vi "duel_ver.vi"() -> ()   [LabVIEW 2024]
uses:
  <vilib>/numeric/Random Number (Range) U64.vi
  <vilib>/numeric/sub_Random U32.vi
panel:
  out "電腦得分":u32
  out "消除數":u16
  out "玩家得分":u32
  out "blocks left":u8
  out "Preview":picture
  in  "Next block":bool
  out "cur block":u8
  out "buf block type":u8[](array[numeric])
  out "rng array":u8[][](array[numeric])
  out "待放置方塊":picture
  in  "direction":enum16{"up", "right", "down", "left"}(ring)
  out "Plate array":u8[][](array[numeric])
  in  "choose_block":u16
  in  "stop":bool
  out "plate":picture
  in  "Turn Block":bool
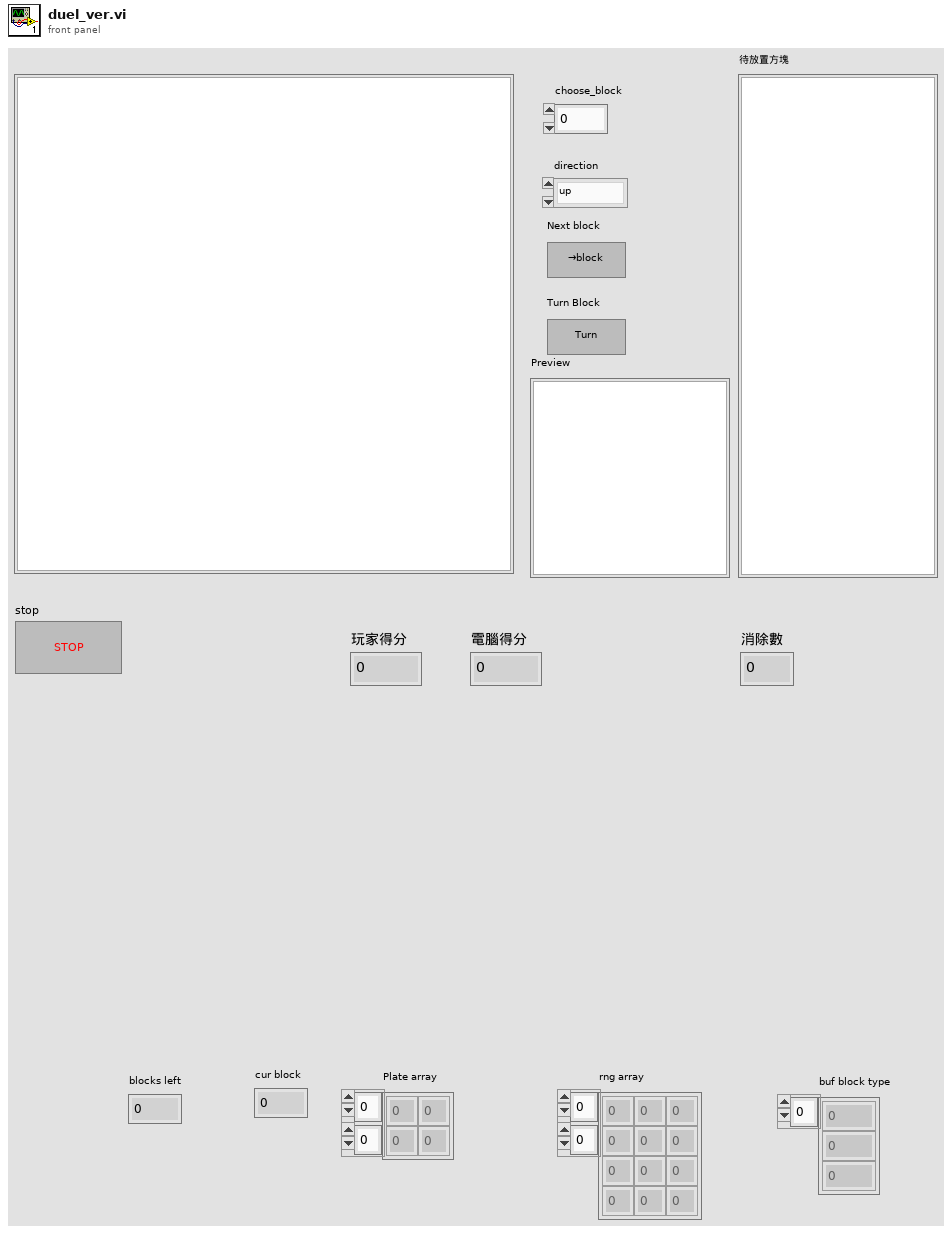
[diagram p1: front panel]
types:
  T1 = typedef "LVPoint32TypeDef.ctl" = cluster{"Horizontal":i32, "Vertical":i32}
  T2 = cluster{"x":u8, "y":u8, "direction":u8, "buf idx":u8}
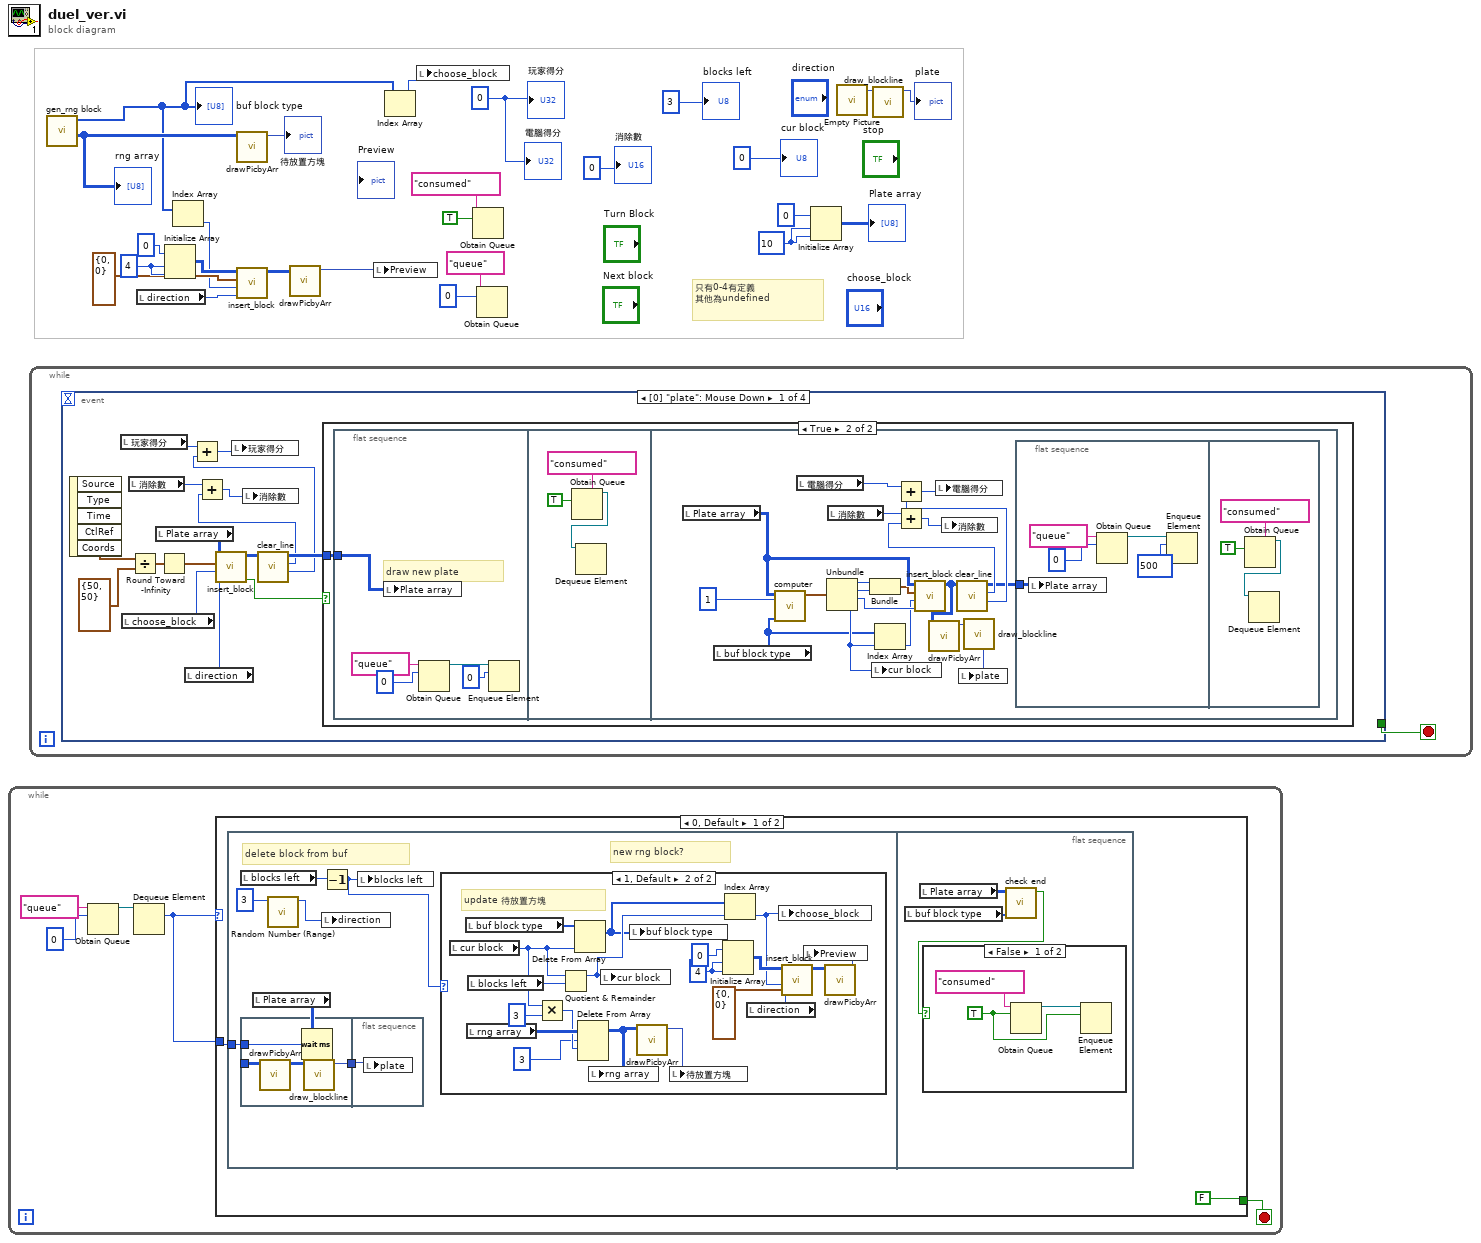
[diagram p0: block diagram]
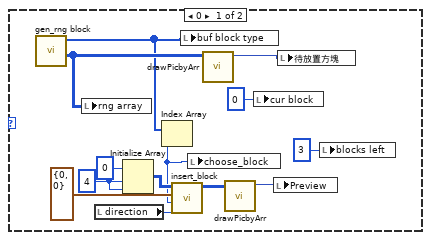
[diagram p2: hidden frame]
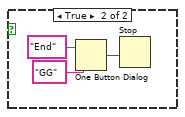
[diagram p3: hidden frame]
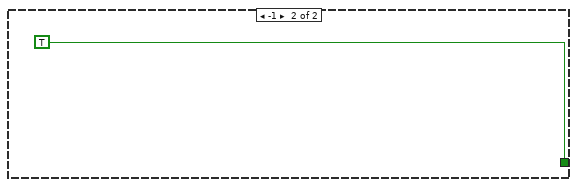
[diagram p4: hidden frame]
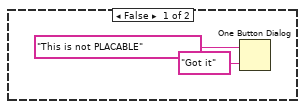
[diagram p5: hidden frame]
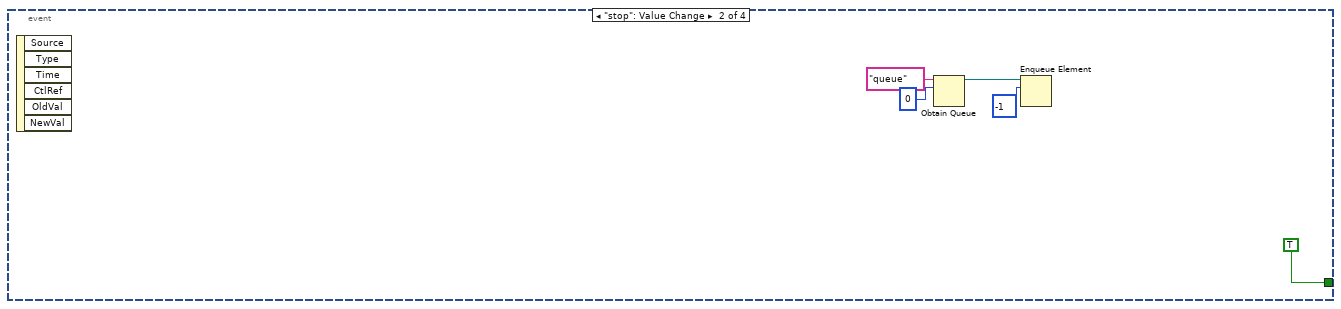
[diagram p6: hidden frame]
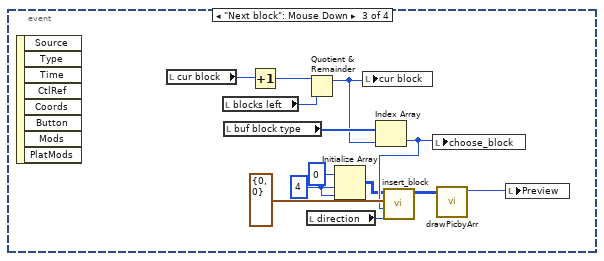
[diagram p7: hidden frame]
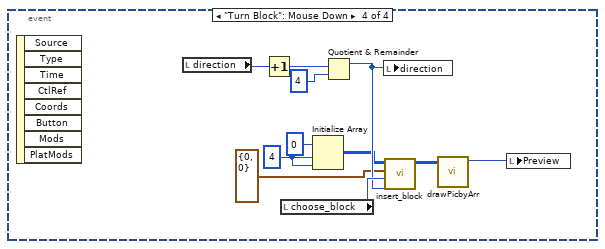
[diagram p8: hidden frame]
diagram:
  w5 = u32 0 ("玩家得分")
  w19 = 4 ("dimension size")
  w23 = 10
  # "只有0-4有定義\n其他為undefined"
  n1 = while {
    stop <- w28 stop-if-true
    n2 = Obtain Queue(name (unnamed)="queue", element data type=0) -> (queue out=w29:refnum<queue>)  [unwired: 3 in, 2 out]
    n3 = Dequeue Element(queue=w29) -> (element=w26:i32)  [unwired: 2 in, 3 out]
    n4 = case shown="0, Default" w26 {
      tunnel: [FALSE TRUE] -> w28
      tunnel: w26 -> [w31 _]
      frame 0, Default {
        n5 = flat-sequence {
          tunnel: w31 -> [w33]
          frame #0 {
            # "new rng block?"
            # "delete block from buf"
            n6 = local read "blocks left"() -> (w36:u8)
            n7 = flat-sequence {
              tunnel: [w74] -> w39
              tunnel: w38 -> [w73]
              tunnel: w33 -> [w72]
              tunnel: w39 -> [w76]
              frame #0 {
                n8 = call "drawPicbyArr.vi"("Array"=w73) -> ("2D Picture"=w75:picture)  [unwired: 10 in]
                n9 = Wait (ms)(milliseconds to wait=w72) -> ()  [unwired: 1 out]
                n10 = call "draw_blockline.vi"("picture in"=w75) -> ("picture out"=w74:picture)  [unwired: 10 in]
              }
              frame #1 {
                n11 = local write "plate"(w76) -> ()
              }
            }
            n12 = local read "Plate array"() -> (w38:u8[][])
            n13 = call-poly <vilib>:"Random Number (Range).vi"("upper bound (100)"=u64 3 ("lower bound (0)")) -> ("number"=w37:u64)  [unwired: 10 in]
            n14 = Decrement(x=w36) -> (x-1=w34:u8)
            n15 = local write "direction"(w37) -> ()
            n16 = local write "blocks left"(w34) -> ()
            n17 = case shown="1, Default" w34 {
              frame 0 {
                w47 = 4 ("dimension size")
                n18 = call "gen_rng block.vi"() -> ("display arr"=w44:u8[][], "Random block"=w40:u8[])  [unwired: 10 in]
                n19 = local write "rng array"(w44) -> ()
                n20 = local read "direction"() -> (w50:enum16{"up", "right", "down", "left"})
                n21 = Initialize Array(u8 0 ("element"), w47, w47) -> (w46:u8[][])
                n22 = Index Array(array=w40) -> (element=w43:u8)  [unwired: 1 in]
                n23 = call "insert_block.vi"("direction"=w50, "block_type"=w43, "position"=cluster{"x":u8, "y":u8} {"x"=0, "y"=0}, "plate arr"=w46) -> ("return plate"=w52:u8[][])  [unwired: 6 in, 1 out]
                n24 = local write "buf block type"(w40) -> ()
                n25 = local write "choose_block"(w43) -> ()
                n26 = call "drawPicbyArr.vi"("Array"=w44) -> ("2D Picture"=w45:picture)  [unwired: 10 in]
                n27 = call "drawPicbyArr.vi"("Array"=w52) -> ("2D Picture"=w51:picture)  [unwired: 10 in]
                n28 = local write "cur block"(u8 0 ("cur block")) -> ()
                n29 = local write "Preview"(w51) -> ()
                n30 = local write "待放置方塊"(w45) -> ()
                n31 = local write "blocks left"(u8 3 ("blocks left")) -> ()
              }
              frame 1, Default {
                w59 = 4 ("dimension size")
                # "update 待放置方塊"
                n32 = local read "cur block"() -> (w56:u8)
                n33 = local read "buf block type"() -> (w71:u8[])
                n34 = local read "rng array"() -> (w70:u8[][])
                n35 = local read "blocks left"() -> (w54:u8)
                n36 = Multiply(x=w56, y=u8 3) -> (x*y=w68:u8)
                n37 = Quotient & Remainder(x=w56, y=w54) -> (x-y*floor(x/y)=w55:u8)  [unwired: 1 out]
                n38 = Delete From Array(array=w71, index=w56) -> (array with subset deleted=w53:u8[])  [unwired: 1 in, 1 out]
                n39 = Delete From Array(array=w70, length=3, index (row)=w68) -> (array with subset deleted=w66:u8[][])  [unwired: 1 in, 1 out]
                n40 = local write "rng array"(w66) -> ()
                n41 = local write "cur block"(w55) -> ()
                n42 = local write "buf block type"(w53) -> ()
                n43 = call "drawPicbyArr.vi"("Array"=w66) -> ("2D Picture"=w65:picture)  [unwired: 10 in]
                n44 = local write "待放置方塊"(w65) -> ()
                n45 = Initialize Array(u8 0 ("element"), w59, w59) -> (w61:u8[][])
                n46 = Index Array(array=w53, index=w55) -> (element=w57:u8)
                n47 = local read "direction"() -> (w62:enum16{"up", "right", "down", "left"})
                n48 = local write "choose_block"(w57) -> ()
                n49 = call "insert_block.vi"("direction"=w62, "block_type"=w57, "position"=cluster{"x":u8, "y":u8} {"x"=0, "y"=0}, "plate arr"=w61) -> ("return plate"=w64:u8[][])  [unwired: 6 in, 1 out]
                n50 = call "drawPicbyArr.vi"("Array"=w64) -> ("2D Picture"=w63:picture)  [unwired: 10 in]
                n51 = local write "Preview"(w63) -> ()
              }
            }
          }
          frame #1 {
            n52 = local read "buf block type"() -> (w78:u8[])
            n53 = local read "Plate array"() -> (w79:u8[][])
            n54 = call "check end.vi"("buf block style"=w78, "input plate"=w79) -> ("End?"=w77:bool)  [unwired: 9 in]
            n55 = case shown="False" w77 {
              frame False {
                w80 = TRUE
                n56 = Obtain Queue(name (unnamed)="consumed", element data type=w80) -> (queue out=w82:refnum<queue>)  [unwired: 3 in, 2 out]
                n57 = Enqueue Element(queue=w82, element=w80) -> ()  [unwired: 2 in, 3 out]
              }
              frame True {
                n58 = One Button Dialog(message="End", button name ("OK")="GG") -> (true=w83:bool)
                n59 = Stop(stop? (T)=w83) -> ()
              }
            }
          }
        }
      }
      frame -1 {
      }
    }
  }
  n60 = while {
    stop <- w87 stop-if-true
    n61 = event shown="[0] \"plate\": Mouse Down" {
      selector: _ -> [_ _ _ _]
      dyn-events: _ -> [_ _ _ _]
      timeout: _ -> [_ _ _ _]
      tunnel: [_ TRUE _ _] -> w87
      event "plate": Mouse Down {
        n62 = event-data() -> ("Coords"=w101:T1)  [unwired: 1 in, 4 out]
        n63 = local read "玩家得分"() -> (w92:u32)
        n64 = local read "choose_block"() -> (w100:u16)
        n65 = local read "消除數"() -> (w93:u16)
        n66 = Divide(x=w101, y=cluster{"Horizontal":u16, "Vertical":u16} {"Horizontal"=50, "Vertical"=50}) -> (x/y=w103:cluster{"Horizontal":dbl, "Vertical":dbl})
        n67 = local read "Plate array"() -> (w99:u8[][])
        n68 = Round Toward -Infinity(1:w103) -> (0:w97:cluster{"Horizontal":dbl, "Vertical":dbl})
        n69 = local read "direction"() -> (w96:enum16{"up", "right", "down", "left"})
        n70 = call "insert_block.vi"("direction"=w96, "block_type"=w100, "position"=w97, "plate arr"=w99) -> ("valid?"=w98:bool, "return plate"=w95:u8[][])  [unwired: 6 in]
        n71 = call "clear_line.vi"("Array in"=w95) -> ("得分"=w90:u32, "消除數"=w91:u8, "Array out"=w94:u8[][])  [unwired: 8 in]
        n72 = Add(x=w92, y=w90) -> (x+y=w89:u32)
        n73 = Add(x=w93, y=w91) -> (x+y=w88:u16)
        n74 = local write "玩家得分"(w89) -> ()
        n75 = local write "消除數"(w88) -> ()
        n76 = case shown="True" w98 {
          tunnel: w94 -> [_ w106]
          frame False {
            n77 = One Button Dialog(message="This is not PLACABLE", button name ("OK")="Got it") -> ()  [unwired: 1 out]
          }
          frame True {
            n78 = flat-sequence {
              tunnel: w106 -> [w111]
              frame #0 {
                # "draw new plate"
                n79 = local write "Plate array"(w111) -> ()
                n80 = Obtain Queue(name (unnamed)="queue", element data type=0) -> (queue out=w110:refnum<queue>)  [unwired: 3 in, 2 out]
                n81 = Enqueue Element(queue=w110, element=0) -> ()  [unwired: 2 in, 3 out]
              }
              frame #1 {
                n82 = Obtain Queue(name (unnamed)="consumed", element data type=TRUE) -> (queue out=w112:refnum<queue>)  [unwired: 3 in, 2 out]
                n83 = Dequeue Element(queue=w112) -> ()  [unwired: 2 in, 4 out]
              }
              frame #2 {
                n84 = local read "Plate array"() -> (w134:u8[][])
                n85 = local read "buf block type"() -> (w119:u8[])
                n86 = call "computer.vi"("buf block style"=w119, "Layer"=u8 1, "input plate"=w134) -> ("record"=w127:T2)  [unwired: 7 in, 1 out]
                n87 = local read "電腦得分"() -> (w123:u32)
                n88 = Unbundle(w127) -> ("x"=w128:u8, "y"=w130:u8, "direction"=w131:u8, "buf idx"=w133:u8)
                n89 = local read "消除數"() -> (w122:u16)
                n90 = Bundle("x"=w128, "y"=w130) -> (w129:cluster{"x":u8, "y":u8})  [unwired: 1 in]
                n91 = local write "cur block"(w133) -> ()
                n92 = Index Array(array=w119, index=w133) -> (element=w120:u8)
                n93 = call "insert_block.vi"("direction"=w131, "block_type"=w120, "position"=w129, "plate arr"=w134) -> ("return plate"=w117:u8[][])  [unwired: 6 in, 1 out]
                n94 = call "drawPicbyArr.vi"("Array"=w117) -> ("2D Picture"=w118:picture)  [unwired: 10 in]
                n95 = call "clear_line.vi"("Array in"=w117) -> ("得分"=w132:u32, "消除數"=w124:u8, "Array out"=w115:u8[][])  [unwired: 8 in]
                n96 = Add(x=w123, y=w132) -> (x+y=w125:u32)
                n97 = Add(x=w122, y=w124) -> (x+y=w126:u16)
                n98 = local write "電腦得分"(w125) -> ()
                n99 = local write "消除數"(w126) -> ()
                n100 = call "draw_blockline.vi"("picture in"=w118) -> ("picture out"=w116:picture)  [unwired: 10 in]
                n101 = local write "plate"(w116) -> ()
                n102 = flat-sequence {
                  tunnel: w115 -> [w139]
                  frame #0 {
                    n103 = local write "Plate array"(w139) -> ()
                    n104 = Obtain Queue(name (unnamed)="queue", element data type=0) -> (queue out=w138:refnum<queue>)  [unwired: 3 in, 2 out]
                    n105 = Enqueue Element(queue=w138, element=500) -> ()  [unwired: 2 in, 3 out]
                  }
                  frame #1 {
                    n106 = Obtain Queue(name (unnamed)="consumed", element data type=TRUE) -> (queue out=w140:refnum<queue>)  [unwired: 3 in, 2 out]
                    n107 = Dequeue Element(queue=w140) -> ()  [unwired: 2 in, 4 out]
                  }
                }
              }
            }
          }
        }
      }
      event "stop": Value Change {
        n108 = event-data() -> ()  [unwired: 1 in, 6 out]
        n109 = Obtain Queue(name (unnamed)="queue", element data type=0) -> (queue out=w145:refnum<queue>)  [unwired: 3 in, 2 out]
        n110 = Enqueue Element(queue=w145, element=-1) -> ()  [unwired: 2 in, 3 out]
      }
      event "Next block": Mouse Down {
        w150 = 4 ("dimension size")
        n111 = event-data() -> ()  [unwired: 1 in, 8 out]
        n112 = local read "cur block"() -> (w160:u8)
        n113 = local read "blocks left"() -> (w148:u8)
        n114 = local read "buf block type"() -> (w158:u8[])
        n115 = Increment(x=w160) -> (x+1=w159:u8)
        n116 = Quotient & Remainder(x=w159, y=w148) -> (x-y*floor(x/y)=w157:u8)  [unwired: 1 out]
        n117 = local read "direction"() -> (w154:enum16{"up", "right", "down", "left"})
        n118 = Initialize Array(u8 0 ("element"), w150, w150) -> (w149:u8[][])
        n119 = local write "cur block"(w157) -> ()
        n120 = Index Array(array=w158, index=w157) -> (element=w152:u8)
        n121 = call "insert_block.vi"("direction"=w154, "block_type"=w152, "position"=cluster{"x":u8, "y":u8} {"x"=0, "y"=0}, "plate arr"=w149) -> ("return plate"=w156:u8[][])  [unwired: 6 in, 1 out]
        n122 = local write "choose_block"(w152) -> ()
        n123 = call "drawPicbyArr.vi"("Array"=w156) -> ("2D Picture"=w155:picture)  [unwired: 10 in]
        n124 = local write "Preview"(w155) -> ()
      }
      event "Turn Block": Mouse Down {
        w162 = 4 ("dimension size")
        n125 = event-data() -> ()  [unwired: 1 in, 8 out]
        n126 = local read "direction"() -> (w168:enum16{"up", "right", "down", "left"})
        n127 = Increment(x=w168) -> (x+1=w169:enum16{"up", "right", "down", "left"})
        n128 = local read "choose_block"() -> (w171:u16)
        n129 = Initialize Array(u8 0 ("element"), w162, w162) -> (w167:u8[][])
        n130 = Quotient & Remainder(x=w169, y=4) -> (x-y*floor(x/y)=w170:i32)  [unwired: 1 out]
        n131 = local write "direction"(w170) -> ()
        n132 = call "insert_block.vi"("direction"=w170, "block_type"=w171, "position"=cluster{"x":u8, "y":u8} {"x"=0, "y"=0}, "plate arr"=w167) -> ("return plate"=w165:u8[][])  [unwired: 6 in, 1 out]
        n133 = call "drawPicbyArr.vi"("Array"=w165) -> ("2D Picture"=w166:picture)  [unwired: 10 in]
        n134 = local write "Preview"(w166) -> ()
      }
    }
  }
  n135 = call "gen_rng block.vi"() -> ("display arr"=w21:u8[][], "Random block"=w11:u8[])  [unwired: 10 in]
  "rng array" <- w21
  "buf block type" <- w11
  n136 = local read "direction"() -> (w16:enum16{"up", "right", "down", "left"})
  n137 = Initialize Array(u8 0 ("element"), w19, w19) -> (w20:u8[][])
  n138 = Index Array(array=w11) -> (element=w13:u8)  [unwired: 1 in]
  n139 = call "drawPicbyArr.vi"("Array"=w21) -> ("2D Picture"=→"待放置方塊":picture)  [unwired: 10 in]
  n140 = call "insert_block.vi"("direction"=w16, "block_type"=w13, "position"=cluster{"x":u8, "y":u8} {"x"=0, "y"=0}, "plate arr"=w20) -> ("return plate"=w14:u8[][])  [unwired: 6 in, 1 out]
  n141 = call "drawPicbyArr.vi"("Array"=w14) -> ("2D Picture"=w15:picture)  [unwired: 10 in]
  n142 = local write "Preview"(w15) -> ()
  n143 = Index Array(array=w11) -> (element=w10:u8)  [unwired: 1 in]
  n144 = local write "choose_block"(w10) -> ()
  n145 = Obtain Queue(name (unnamed)="consumed", element data type=TRUE) -> ()  [unwired: 3 in, 3 out]
  n146 = Obtain Queue(name (unnamed)="queue", element data type=0) -> ()  [unwired: 3 in, 3 out]
  n147 = Initialize Array(u8 0 ("element"), w23, w23) -> (→"Plate array":u8[][])
  n148 = call "Empty Picture"() -> ("empty picture"=w8:picture)
  n149 = call "draw_blockline.vi"("picture in"=w8) -> ("picture out"=→"plate":picture)  [unwired: 10 in]
  "cur block" <- 0
  "blocks left" <- u8 3 ("blocks left")
  "玩家得分" <- w5
  "消除數" <- u16 0 ("消除數")
  "電腦得分" <- w5
